vi "HXG2_Timing Module Blower.vi"(7 "Timer Command":T1=enum."Start", 8 "error in (no error)":errorcluster) -> (0 "error out":errorcluster, 1 "Elapsed Time":dbl, 2 "Done?":bool)   [LabVIEW 2012]
doc: "This VI is a functional global variable that keeps track the amount of time elapsed since a Start command was sent to the VI."
uses:
  HXG2_BlowerPumpl.ctl
panel:
  # "Input"
  # "Output"
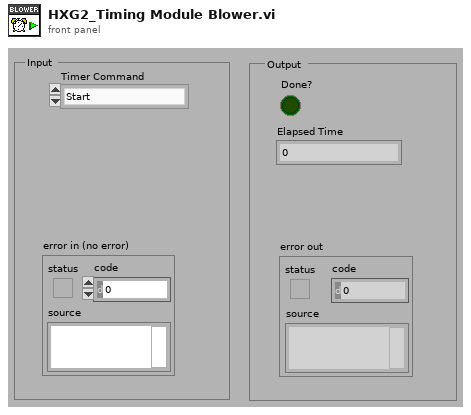
[diagram p1: front panel]
types:
  T1 = typedef "HXG2_BlowerPumpl.ctl" = enum16{"Stop", "Start", "Check Time"}
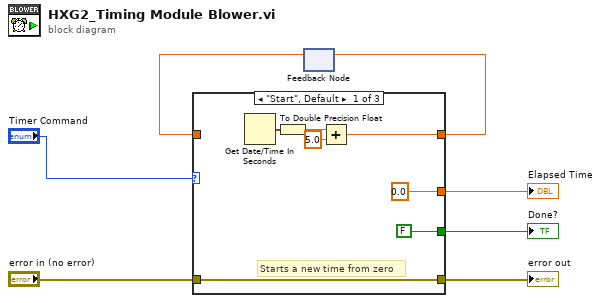
[diagram p0: block diagram]
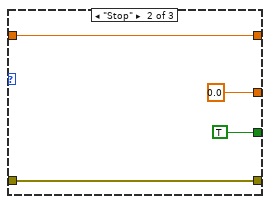
[diagram p2: hidden frame]
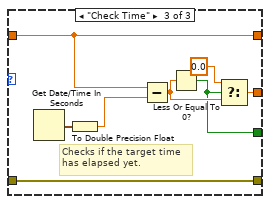
[diagram p3: hidden frame]
diagram:
  n1 = feedback #1() -> (w3:dbl)  [unwired: 1 in]
  n2 = case shown="\"Start\", Default" "Timer Command" {
    tunnel: [w8 w15 w20] -> w4
    tunnel: w3 -> [_ w15 w20]
    tunnel: [0.0 ("double precision float") 0.0 ("double precision float") w24] -> w7
    tunnel: [FALSE TRUE w21] -> w6
    tunnel: "error in (no error)" -> [w11 w16 w25]
    tunnel: [w11 w16 w25] -> w1
    frame "Start", Default {
      # "Starts a new time from zero"
      n3 = Get Date/Time In Seconds() -> (seconds since 1Jan1904=w14:timestamp)
      n4 = To Double Precision Float(number=w14) -> (double precision float=w10:dbl)
      n5 = Add(x=w10, y=5.0) -> (x+y=w8:dbl)
    }
    frame "Stop" {
    }
    frame "Check Time" {
      # "Checks if the target time\nhas elapsed yet."
      n6 = Get Date/Time In Seconds() -> (seconds since 1Jan1904=w26:timestamp)
      n7 = To Double Precision Float(number=w26) -> (double precision float=w19:dbl)
      n8 = Subtract(x=w20, y=w19) -> (x-y=w22:dbl)
      n9 = Less Or Equal To 0?(x=w22) -> (x <= 0?=w21:bool)
      n10 = Select(t=0.0, s=w21, f=w22) -> (s? t:f=w24:dbl)
    }
  }
  "error out" <- w1
  "Elapsed Time" <- w7
  "Done?" <- w6
  n11 = feedback-in #1(w4) -> ()
